vi "Migrate Measurements.vi"() -> ()   [LabVIEW 2021]
uses:
  _Measurement Plugin Converter/Migrator/Queue Driver/controls/Queue Operations.ctl
  _Measurement Plugin Converter/Migrator/Migration Logic/controls/Multiple Migration/Multiple Migration Data Holder.ctl
  <vilib>/Utility/sysdir.llb/System Directory Type.ctl
  <vilib>/Utility/miscctls.llb/LVRowAndColumnUnsignedTypeDef.ctl
  <vilib>/Utility/miscctls.llb/LVRowAndColumnTypeDef.ctl
  _Measurement Plugin Converter/Migrator/Migrator Reusables/controls/Dictionary States.ctl
  <vilib>/Utility/cursorutil.llb/Set Cursor (Icon Pict).vi
  _Measurement Plugin Converter/Migrator/Queue Driver/Queue Driver.lvlib
  _Measurement Plugin Converter/Migrator/Migration Logic/Migrator.lvlib
  _Measurement Plugin Converter/Migrator/Path Functions/Path Functions.lvlib
  _Measurement Plugin Converter/Migrator/Multiple Migrator/Multiple Migrator.lvlib
  _Measurement Plugin Converter/Migrator/Migrator Reusables/Migrator Reusables.lvlib
panel:
  out "error out":errorcluster
  in  "Tab Control":T1(tab)
  in  "Info":string
  in  "Select Measurement":path
  out "Warning":bool=TRUE caption="Warning:\nMeasurement should be an existing VI or folder path"
  in  "Populate measurements":bool
  in  "Select Project":path
  in  "Select all":bool
  in  "Back to Home":bool
  in  "List Plug-ins":bool
  in  "Select Measurements":string(tree)
  out "Selection warning":string="Atleast one measurement should be selected"
  out "Plug-in info":string="* Rename the Plug-in if required"
  out "Plug-in warning":string="Warning:\n1. Measurement plug-in name must be unique \n2. Plugin name cannot contain any of the following characters:\n         \\ / : * ? \" < > |"
  in  "Start Migration":bool
  in  "Back to Select":bool
  in  "List of Selected Measurements":i32(listbox)
  in  "Measurement Count":i32(slide)=6 caption="Migrating 1 of 1 measurement(s)" scale=0.0..100.0
  in  "Progress":i32(slide)=9 caption="Saving the project files..." scale=0.0..15.0
  in  "Review":bool
  in  "Migration Status":i32(listbox)
  in  "Back to Status":bool
  in  "Select Plug-in":string(combo) caption="Select Measurement plug-in to review"
  in  "Start Next":bool
  out "Launch Type Spec":string
  out "Launch Logic":string
  out "Launch UI":string
  # "* Project in which the measurement plug-in will be created"
  # "* Select a measurement vi or a folder containing measurements"
  # ".lvproj"
  # "Select the measurements to migrate"
  # "Review the Measurement:\n1. Review the Measurement UI. Click here to launch.\n2. Review the Measurement Logic VI. Click here to launch.\n3. Review the Type Specialization VI. Click here to launch."
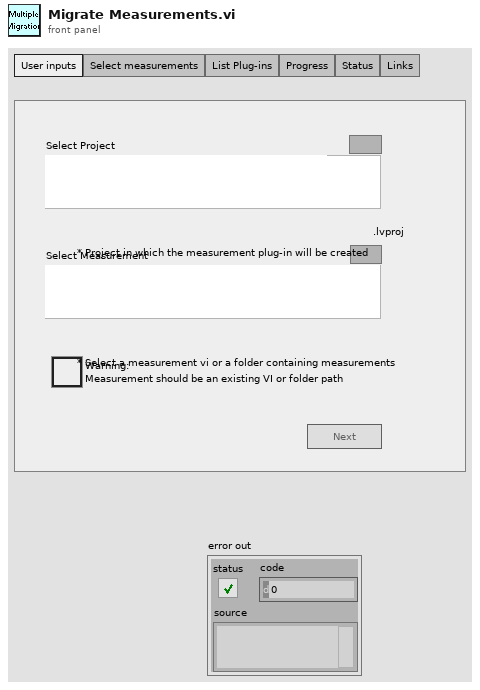
[diagram p1: front panel]
types:
  T1 = enum32{"User inputs", "Select measurements", "List Plug-ins", "Progress", "Status", "Links"}
  T2 = typedef "Queue Driver.lvlib/Queue Operations.ctl" = enum16{"Create Q", "Enqueue", "Enqueue N", "Dequeue", "Flush", "Release"}
  T3 = typedef "Migrator.lvlib/Multiple Migration Data Holder.ctl" = cluster{"Tree Reference":refnum<vi>, "LabVIEW Version":string, "Project path":path, "Create new project?":bool, "Measurement file/folder path":path, "Measurement folder selected?":bool, "Project warning":string, "Measurement warning":string, "Next clicked?":bool, "Measurement path changed?":bool, "Select all":bool, "Measurement folder Tags":string[], "Measurement file Tags":string[], "Selected cell Tag":string, "Measurement Plug-ins":string[][], "Measurement File Paths":path[], "Plugin Migration Value":i32, "Migration Count":i32, "Instrument containing subVIs":path[][], "Progress per measurement":i32, "Measurement Progress":i32, "Migration Status":string[][]}
  T4 = enum8{"Enabled", "Disabled", "Disabled and Grayed Out"}
  T5 = typedef "LVRowAndColumnUnsignedTypeDef.ctl" = cluster{"Row":u32, "Column":u32}
  T6 = typedef "LVRowAndColumnTypeDef.ctl" = cluster{"Row":i32, "Column":i32}
  T7 = typedef "Migrator Reusables.lvlib/Dictionary States.ctl" = enum16{"Set", "Get", "Delete", "Delete All"}
  T8 = typedef "System Directory Type.ctl" = i32
  T9 = typedef "LVPoint32TypeDef.ctl" = cluster{"Horizontal":i32, "Vertical":i32}
  T10 = typedef "Migrator.lvlib/Tree Items.ctl" = cluster{"Item name":string, "Indent":i32, "Tag":string}
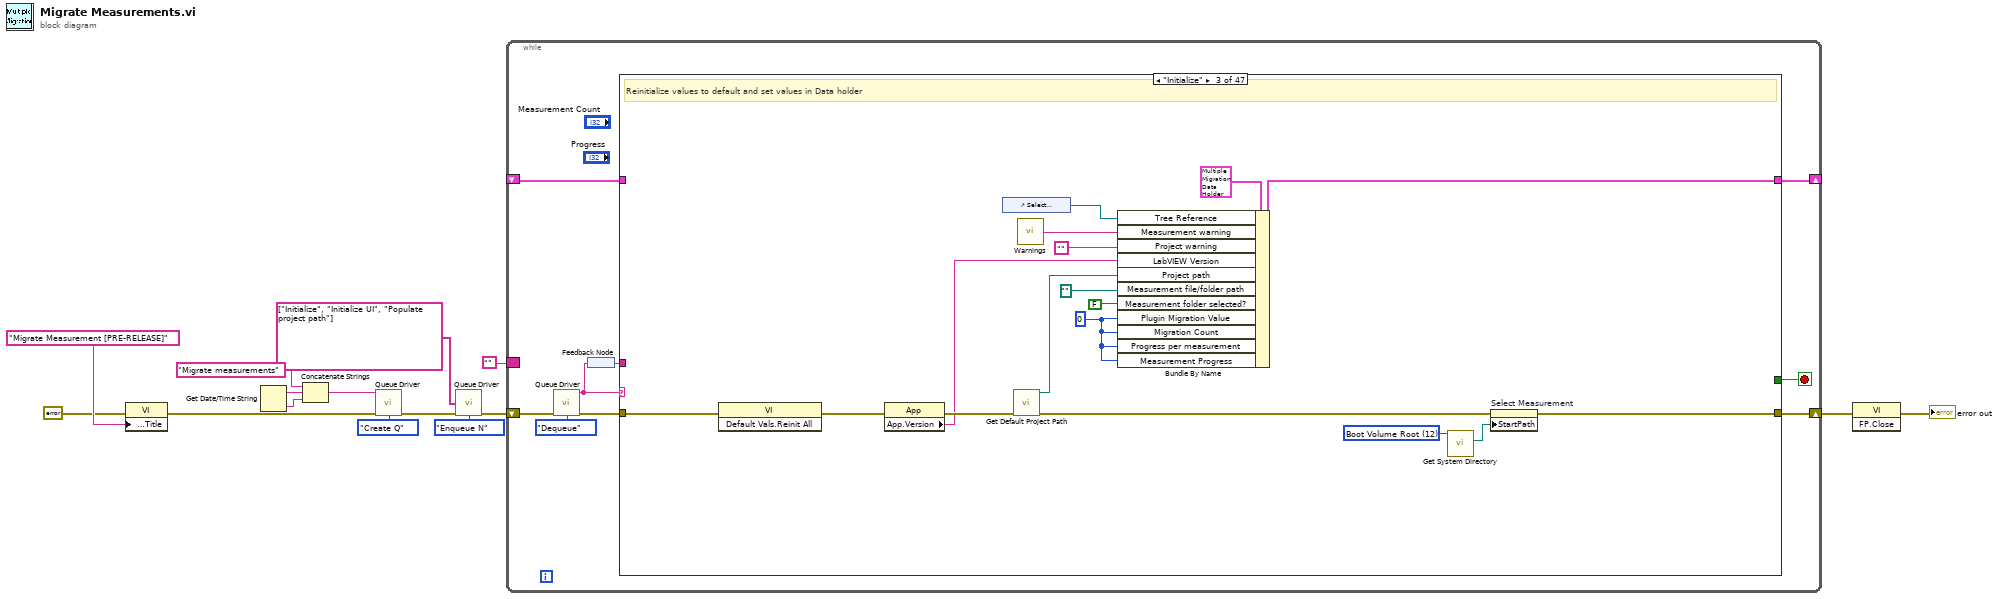
[diagram p0: block diagram]
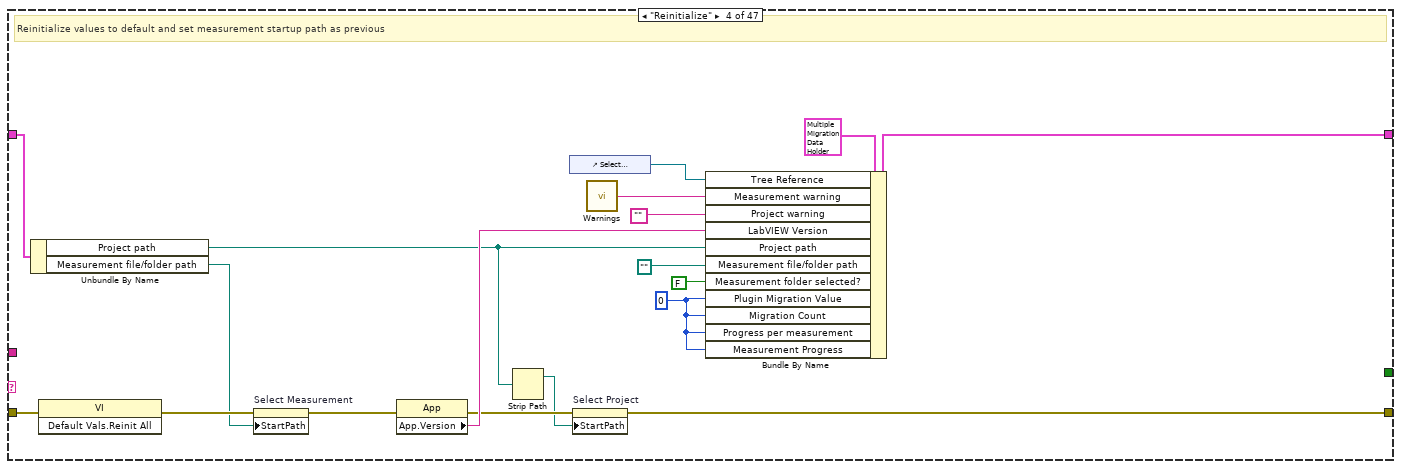
[diagram p4: hidden frame]
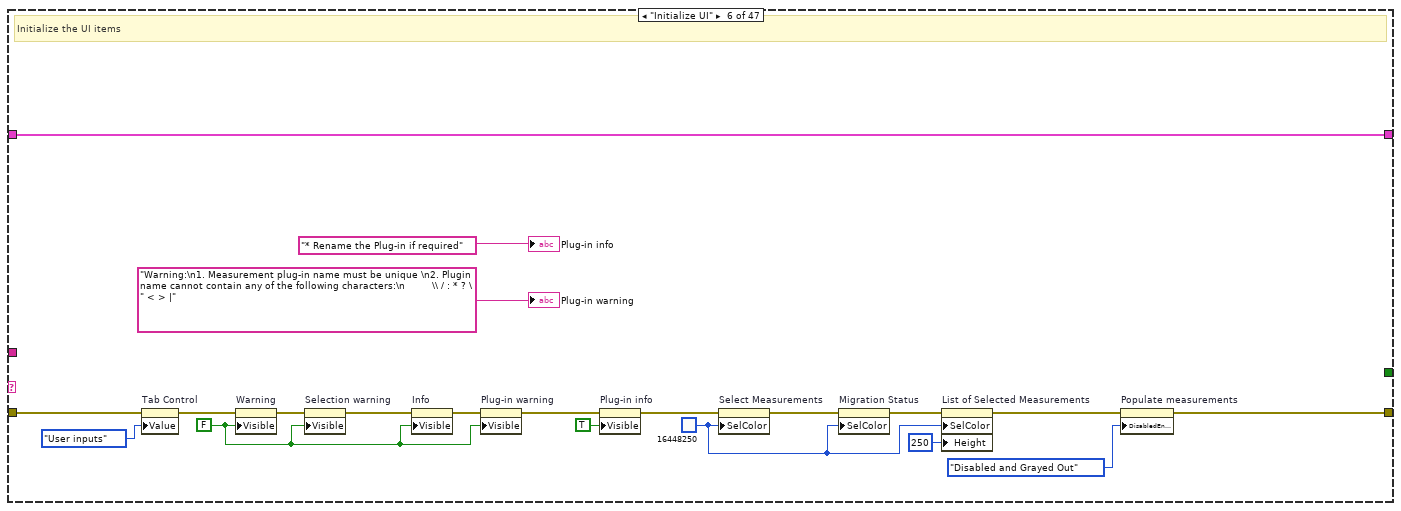
[diagram p6: hidden frame]
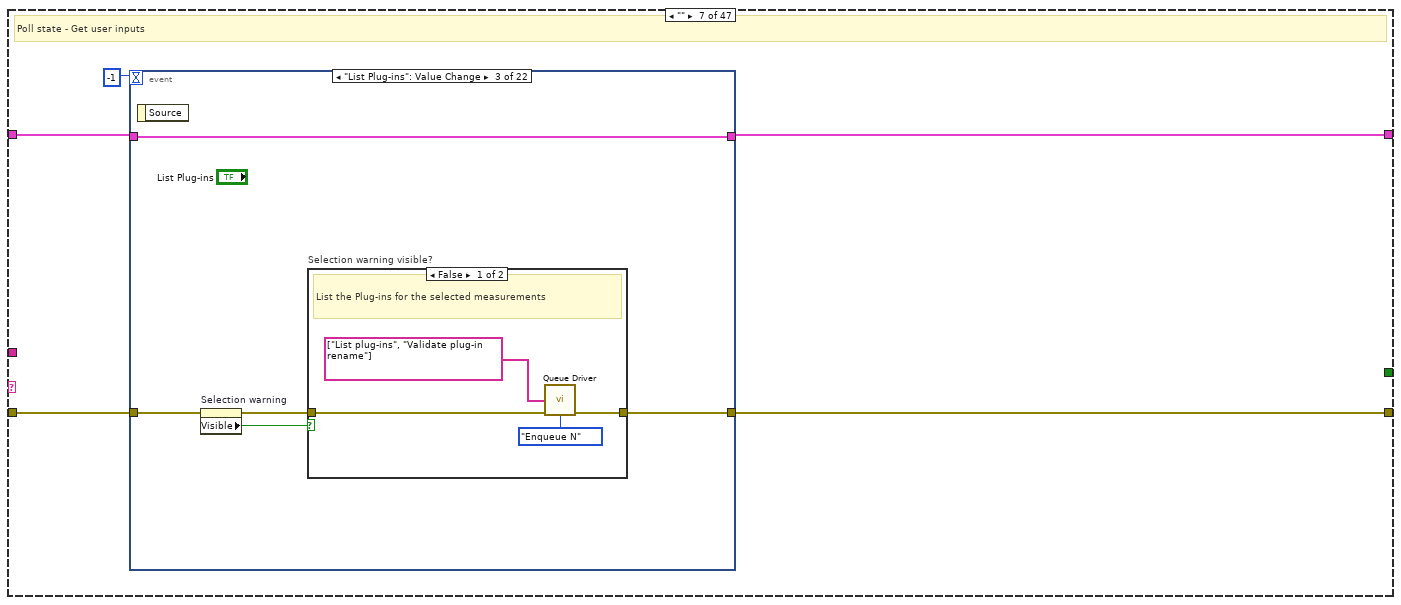
[diagram p7: hidden frame]
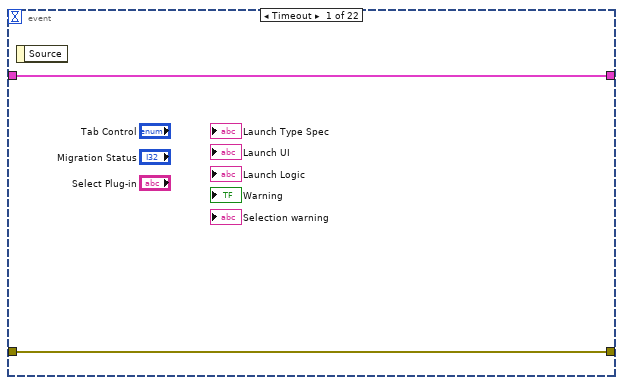
[diagram p8: hidden frame]
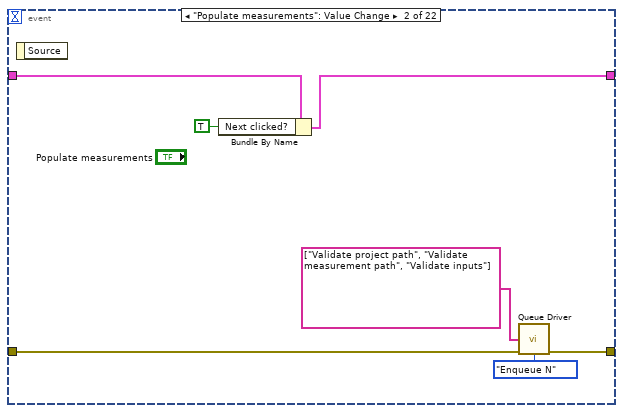
[diagram p9: hidden frame]
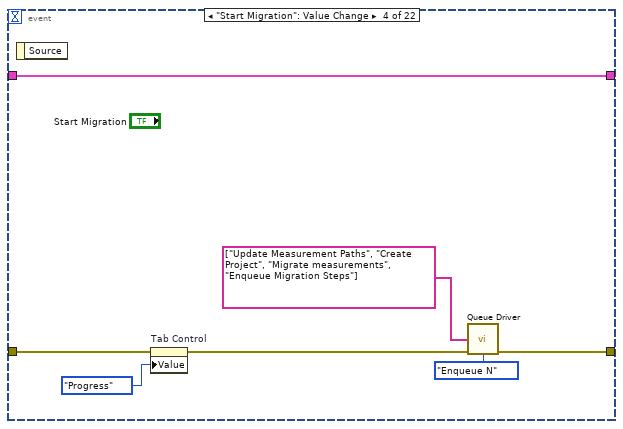
[diagram p11: hidden frame]
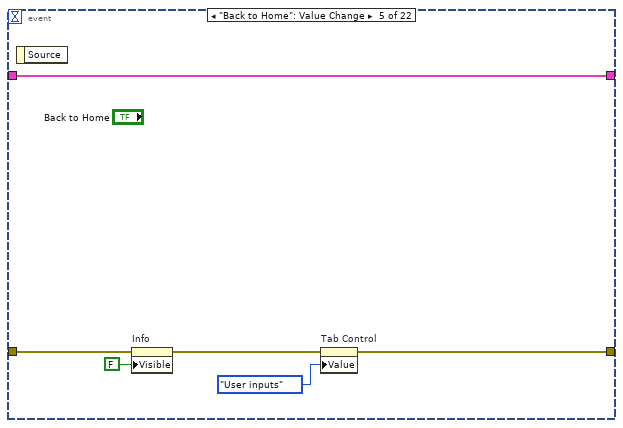
[diagram p12: hidden frame]
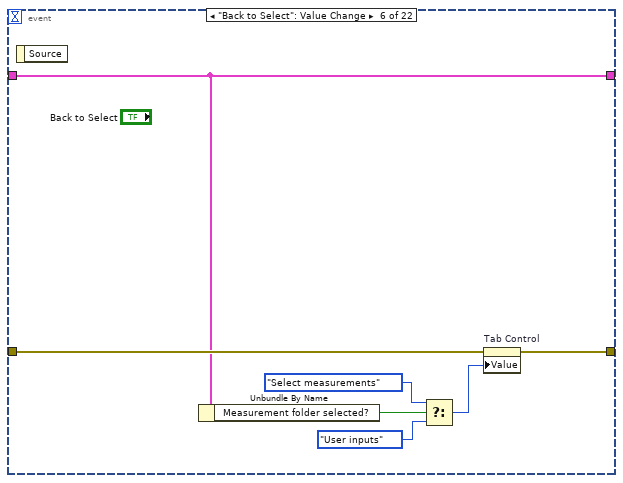
[diagram p13: hidden frame]
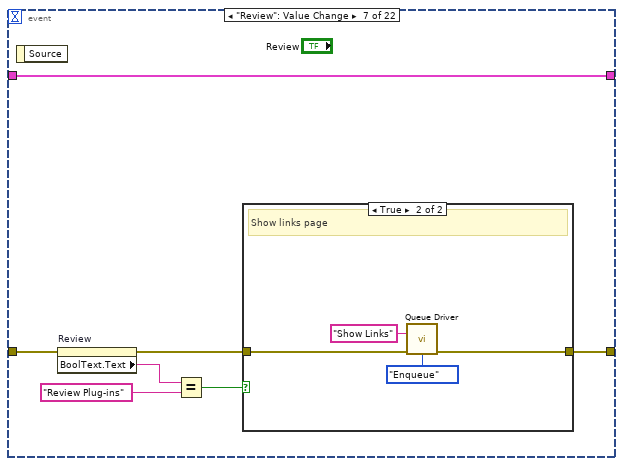
[diagram p14: hidden frame]
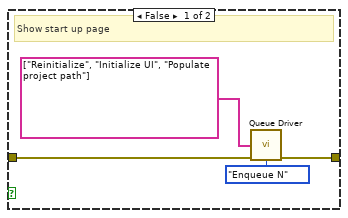
[diagram p15: hidden frame]
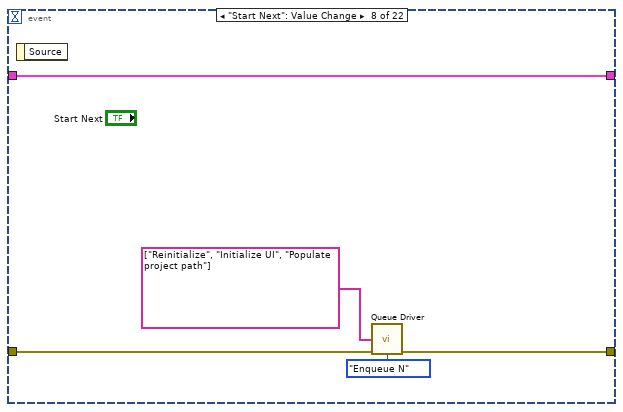
[diagram p16: hidden frame]
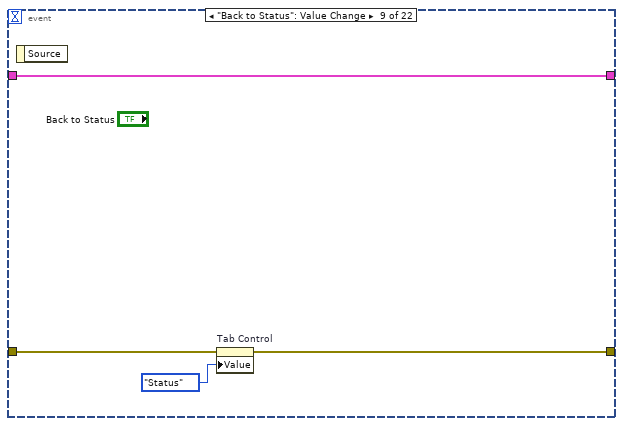
[diagram p17: hidden frame]
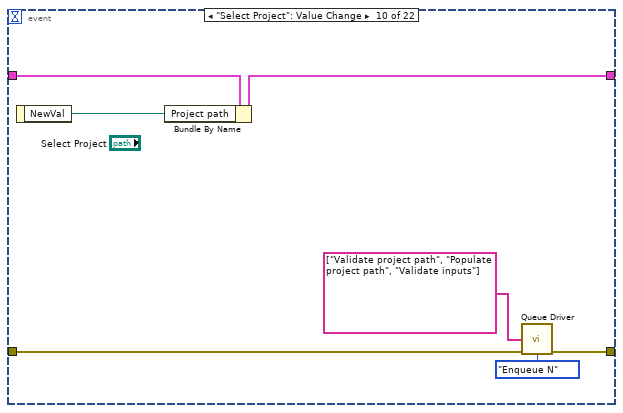
[diagram p18: hidden frame]
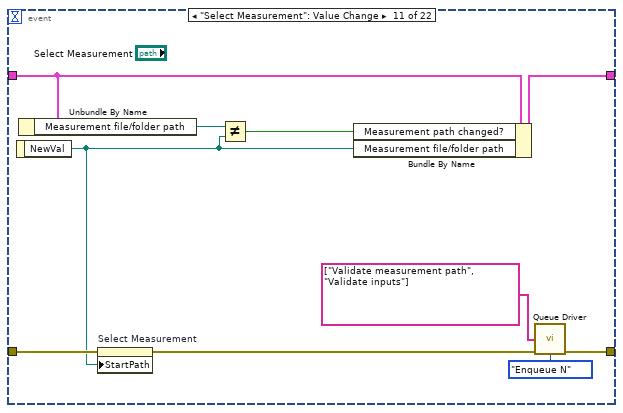
[diagram p19: hidden frame]
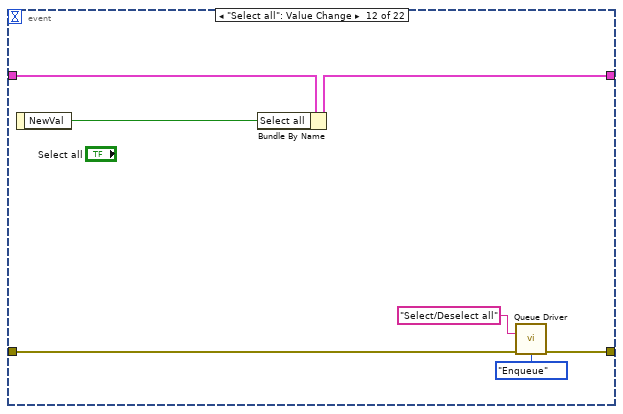
[diagram p20: hidden frame]
diagram:
  n1 = property class="VI"(error in=errorcluster {"status"=FALSE, "code"=0, "source"=""} ("error in (no error)"), "Front Panel.Title"="Migrate Measurement [PRE-RELEASE]" ("Front Panel Window:Title")) -> (error out=w1:errorcluster)  [unwired: 1 in, 1 out]
  n2 = Get Date/Time String() -> (date string=w12:string, time string=w11:string)  [unwired: 3 in]
  n3 = Concatenate Strings("Migrate measurements" ("string"), w12, w11) -> (w7:string)
  n4 = call "Queue Driver.vi"("Name"=w7, "error in (no error)"=w1, "Q Operations"=Queue_Operations."Create Q") -> ("error out"=w15:errorcluster)  [unwired: 11 in, 1 out]
  n5 = call "Queue Driver.vi"("States[]"=string[] ["Initialize", "Initialize UI", "Populate project path"], "error in (no error)"=w15, "Q Operations"=Queue_Operations."Enqueue N") -> ("error out"=w10:errorcluster)  [unwired: 11 in, 1 out]
  n6 = while {
    shift-right: [w23] -> w6
    shift-left: w10 -> [w24]
    shift-right: [w20] -> _
    shift-left: _ -> [w19]
    border: "" -> [_]
    stop <- w18 stop-if-true
    n7 = call "Queue Driver.vi"("error in (no error)"=w24, "Q Operations"=Queue_Operations."Dequeue") -> ("Dequeued State"=w17:string, "error out"=w22:errorcluster)  [unwired: 12 in]
    n8 = feedback #1() -> (w16:string)
    n9 = feedback-in #1(w17) -> ()
    n10 = case shown="\"Initialize\"" w17 {
      tunnel: w22 -> [w25 w28 w45 w63 w65 w85 w90 w262 w274 w285 w304 w328 w377 w394 w447 w472 w491 w548 w558 w564 w587 w597 w616 w633 w655 w662 w668 w674 w680 w686 w692 w698 w704 w710 w716 w722 w728 w734 w740 w762 w783 w795 w837 w846 w855 w876 w888]
      tunnel: [w25 w28 w34 w48 w65 w76 w89 w264 w274 w277 w303 w327 w377 w389 w435 w455 w478 w538 w558 w559 w584 w600 w615 w632 w654 w664 w670 w676 w682 w688 w694 w700 w706 w712 w718 w724 w730 w735 w744 w766 w783 w794 w834 w846 w852 w876 w878] -> w23
      tunnel: [w26 w27 w44 w62 w64 w81 w86 w263 w275 w280 w297 w315 w378 w395 w438 w470 w475 w543 w557 w579 w595 w609 w619 w652 w660 w666 w672 w678 w684 w690 w696 w702 w708 w714 w720 w726 w732 w738 w745 w767 w784 w799 w836 w847 w857 w877 w886] -> w20
      tunnel: w19 -> [w26 w27 _ w51 w64 w81 w87 w263 w275 w281 w299 w326 w378 w396 w439 w471 w476 w544 w557 w580 w595 w608 w619 w652 w660 w666 w672 w678 w684 w690 w696 w702 w708 w714 w720 w726 w732 w738 w746 w768 w784 w800 w836 w847 w857 w877 w886]
      tunnel: [_ _ _ _ _ _ _ _ _ _ _ _ _ _ _ _ _ _ _ _ _ _ _ _ _ _ _ _ _ _ _ _ _ _ _ _ _ _ _ _ _ _ _ _ _ _ TRUE] -> w18
      tunnel: w16 -> [_ _ _ _ _ _ _ _ _ _ _ _ _ _ _ _ _ _ _ _ _ _ _ _ _ _ _ _ _ _ _ _ _ _ _ _ _ _ _ _ _ _ _ _ w848 _ _]
      frame Default {
        # "Default case"
      }
      frame "/**********INITIALIZE**********/" {
      }
      frame "Initialize" {
        w29 = 0 ("Plugin Migration Value")
        w33 = T8 12 items=["User Home"=0, "User Desktop"=1, "User Documents"=2, "User Application Data"=3, "User Preferences"=4, "User Temporary"=5, "Public Documents"=6, "Public Application Data"=7, "Public Preferences"=8, "Public Cache"=13, "System Core Libraries"=9, "System Installed Libraries"=10, "Application Files"=11, "Boot Volume Root"=12] ("system directory type")
        # "Reinitialize values to default and set values in Data holder"
        n11 = invoke class="VI" method="Default Vals.Reinit All"(error in=w45) -> (error out=w42:errorcluster)  [unwired: 2 in, 2 out]
        n12 = property class="App"(error in=w42) -> (error out=w41:errorcluster, "App.Version"=w40:string)  [unwired: 1 in, 1 out]
        n13 = control-ref of="Select Measurements"() -> (w37:refnum<vi>)
        n14 = call "Get Default Project Path.vi"("error in"=w41) -> ("Project Path"=w43:path, "error out"=w35:errorcluster)  [unwired: 13 in]
        n15 = call "Warnings.vi"() -> ("Invalid measurement path"=w36:string)  [unwired: 8 in, 7 out]
        n16 = Bundle By Name(cluster=T3 {"Tree Reference"=refnum, "LabVIEW Version"="", "Project path"=path "", "Create new project?"=FALSE, "Measurement file/folder path"=path "", "Measurement folder selected?"=FALSE, "Project warning"="", "Measurement warning"="", "Next clicked?"=FALSE, "Measurement path changed?"=FALSE, "Select all"=FALSE, "Measurement folder Tags"=[], "Measurement file Tags"=[], "Selected cell Tag"="", "Measurement Plug-ins"=[], "Measurement File Paths"=[], "Plugin Migration Value"=0, "Migration Count"=0, "Instrument containing subVIs"=[], "Progress per measurement"=0, "Measurement Progress"=0, "Migration Status"=[]}, "Tree Reference"=w37, "Measurement warning"=w36, "Project warning"="", "LabVIEW Version"=w40, "Project path"=w43, "Measurement file/folder path"=path "", "Measurement folder selected?"=FALSE, "Plugin Migration Value"=w29, "Migration Count"=w29, "Progress per measurement"=w29, "Measurement Progress"=w29) -> (w44:T3)
        n17 = call <vilib>:"Get System Directory.vi"("system directory type"=w33) -> ("system directory"=w32:path)  [unwired: 10 in]
        n18 = property on="Select Measurement" class="Path"(error in=w35, "StartPath"=w32) -> (error out=w34:errorcluster)  [unwired: 1 in, 1 out]
      }
      frame "Reinitialize" {
        w54 = 0 ("Plugin Migration Value")
        # "Reinitialize values to default and set measurement startup path as previous"
        n19 = Unbundle By Name(w51) -> ("Project path"=w47:path, "Measurement file/folder path"=w50:path)
        n20 = invoke class="VI" method="Default Vals.Reinit All"(error in=w63) -> (error out=w53:errorcluster)  [unwired: 2 in, 2 out]
        n21 = property on="Select Measurement" class="Path"(error in=w53, "StartPath"=w50) -> (error out=w52:errorcluster)  [unwired: 1 in, 1 out]
        n22 = property class="App"(error in=w52) -> (error out=w49:errorcluster, "App.Version"=w61:string)  [unwired: 1 in, 1 out]
        n23 = Strip Path(path=w47) -> (stripped path=w46:path)  [unwired: 1 out]
        n24 = control-ref of="Select Measurements"() -> (w58:refnum<vi>)
        n25 = property on="Select Project" class="Path"(error in=w49, "StartPath"=w46) -> (error out=w48:errorcluster)  [unwired: 1 in, 1 out]
        n26 = call "Warnings.vi"() -> ("Invalid measurement path"=w57:string)  [unwired: 8 in, 7 out]
        n27 = Bundle By Name(cluster=T3 {"Tree Reference"=refnum, "LabVIEW Version"="", "Project path"=path "", "Create new project?"=FALSE, "Measurement file/folder path"=path "", "Measurement folder selected?"=FALSE, "Project warning"="", "Measurement warning"="", "Next clicked?"=FALSE, "Measurement path changed?"=FALSE, "Select all"=FALSE, "Measurement folder Tags"=[], "Measurement file Tags"=[], "Selected cell Tag"="", "Measurement Plug-ins"=[], "Measurement File Paths"=[], "Plugin Migration Value"=0, "Migration Count"=0, "Instrument containing subVIs"=[], "Progress per measurement"=0, "Measurement Progress"=0, "Migration Status"=[]}, "Tree Reference"=w58, "Measurement warning"=w57, "Project warning"="", "LabVIEW Version"=w61, "Project path"=w47, "Measurement file/folder path"=path "", "Measurement folder selected?"=FALSE, "Plugin Migration Value"=w54, "Migration Count"=w54, "Progress per measurement"=w54, "Measurement Progress"=w54) -> (w62:T3)
      }
      frame "/**********FP RELATED**********/" {
      }
      frame "Initialize UI" {
        w70 = FALSE ("Visible")
        w78 = u32 16448250 ("Selection Color")
        # "Initialize the UI items"
        n28 = property on="Tab Control" class="TabCtl (strict)"(error in=w85, "Value"=T1."User inputs" ("Tab Control")) -> (error out=w80:errorcluster)  [unwired: 1 in, 1 out]
        n29 = property on="Warning" class="Bool"(error in=w80, "Visible"=w70) -> (error out=w79:errorcluster)  [unwired: 1 in, 1 out]
        n30 = property on="Selection warning" class="Str"(error in=w79, "Visible"=w70) -> (error out=w74:errorcluster)  [unwired: 1 in, 1 out]
        n31 = property on="Info" class="Str"(error in=w74, "Visible"=w70) -> (error out=w73:errorcluster)  [unwired: 1 in, 1 out]
        n32 = property on="Plug-in warning" class="Str"(error in=w73, "Visible"=w70) -> (error out=w69:errorcluster)  [unwired: 1 in, 1 out]
        n33 = property on="Plug-in info" class="Str"(error in=w69, "Visible"=TRUE) -> (error out=w68:errorcluster)  [unwired: 1 in, 1 out]
        n34 = property on="Select Measurements" class="Tree (strict)"(error in=w68, "SelColor"=w78) -> (error out=w83:errorcluster)  [unwired: 1 in, 1 out]
        n35 = property on="Migration Status" class="MCListbox (strict)"(error in=w83, "SelColor"=w78) -> (error out=w82:errorcluster)  [unwired: 1 in, 1 out]
        n36 = property on="List of Selected Measurements" class="MCListbox (strict)"(error in=w82, "SelColor"=w78, "Height"=u32 250 ("Size:Height")) -> (error out=w77:errorcluster)  [unwired: 1 in, 1 out]
        n37 = property on="Populate measurements" class="Bool"(error in=w77, "DisabledEnum"=T4."Disabled and Grayed Out" ("Disabled")) -> (error out=w76:errorcluster)  [unwired: 1 in, 1 out]
        "Plug-in warning" <- "Warning:\n1. Measurement plug-in name must be unique \n2. Plugin name cannot contain any of the following characters:\n         \\ / : * ? \" < > |" ("f")
        "Plug-in info" <- "* Rename the Plug-in if required" ("Plug-in warning")
      }
      frame "" {
        # "Poll state - Get user inputs"
        n38 = event shown="[2] \"List Plug-ins\": Value Change" {
          selector: _ -> [_ _ _ _ _ _ _ _ _ _ _ _ _ _ _ _ _ _ _ _ _ _]
          dyn-events: _ -> [_ _ _ _ _ _ _ _ _ _ _ _ _ _ _ _ _ _ _ _ _ _]
          timeout: -1 -> [_ _ _ _ _ _ _ _ _ _ _ _ _ _ _ _ _ _ _ _ _ _]
          tunnel: w90 -> [w92 w99 w102 w116 w119 w129 w133 w146 w153 w160 w166 w174 w185 w194 w202 w209 w212 w216 w222 w232 w244 w256]
          tunnel: [w92 w98 w103 w112 w122 w128 w135 w147 w152 w159 w169 w173 w180 w193 w200 w210 w213 w217 w224 w235 w246 w255] -> w89
          tunnel: w87 -> [w91 w95 w104 w113 w120 w127 w136 w149 w150 w157 w164 w177 w184 w195 w203 w211 w215 w219 w225 w236 w247 w257]
          tunnel: [w91 w94 w104 w113 w120 w127 w136 w149 w150 w156 w170 w176 w183 w195 w203 w211 w215 w219 w225 w236 w247 w257] -> w86
          event Timeout {
            # "Timeout"
            n39 = event-data() -> ()  [unwired: 1 in, 1 out]
          }
          event "Populate measurements": Value Change {
            n40 = event-data() -> ()  [unwired: 1 in, 1 out]
            n41 = Bundle By Name(cluster=w95, "Next clicked?"=TRUE) -> (w94:T3)
            n42 = call "Queue Driver.vi"("States[]"=string[] ["Validate project path", "Validate measurement path", "Validate inputs"], "error in (no error)"=w99, "Q Operations"=Queue_Operations."Enqueue N") -> ("error out"=w98:errorcluster)  [unwired: 11 in, 1 out]
          }
          event "List Plug-ins": Value Change {
            n43 = event-data() -> ()  [unwired: 1 in, 1 out]
            n44 = property on="Selection warning" class="Str"(error in=w102) -> (error out=w101:errorcluster, "Visible"=w100:bool)  [unwired: 1 in, 1 out]
            n45 = case "Selection warning visible?" shown="False" w100 {
              tunnel: w101 -> [w108 w109]
              tunnel: [w107 w109] -> w103
              frame False {
                # "List the Plug-ins for the selected measurements"
                n46 = call "Queue Driver.vi"("States[]"=string[] ["List plug-ins", "Validate plug-in rename"], "error in (no error)"=w108, "Q Operations"=Queue_Operations."Enqueue N") -> ("error out"=w107:errorcluster)  [unwired: 11 in, 1 out]
              }
              frame True {
                # "Pass"
              }
            }
          }
          event "Start Migration": Value Change {
            n47 = event-data() -> ()  [unwired: 1 in, 1 out]
            n48 = property on="Tab Control" class="TabCtl (strict)"(error in=w116, "Value"=T1."Progress" ("Tab Control")) -> (error out=w115:errorcluster)  [unwired: 1 in, 1 out]
            n49 = call "Queue Driver.vi"("States[]"=string[] ["Update Measurement Paths", "Create Project", "Migrate measurements", "Enqueue Migration Steps"], "error in (no error)"=w115, "Q Operations"=Queue_Operations."Enqueue N") -> ("error out"=w112:errorcluster)  [unwired: 11 in, 1 out]
          }
          event "Back to Home": Value Change {
            n50 = event-data() -> ()  [unwired: 1 in, 1 out]
            n51 = property on="Info" class="Str"(error in=w119, "Visible"=FALSE) -> (error out=w118:errorcluster)  [unwired: 1 in, 1 out]
            n52 = property on="Tab Control" class="TabCtl (strict)"(error in=w118, "Value"=T1."User inputs" ("Tab Control")) -> (error out=w122:errorcluster)  [unwired: 1 in, 1 out]
          }
          event "Back to Select": Value Change {
            n53 = event-data() -> ()  [unwired: 1 in, 1 out]
            n54 = Unbundle By Name(w127) -> ("Measurement folder selected?"=w126:bool)
            n55 = Select(t=T1."Select measurements" ("Tab Control"), s=w126, f=T1."User inputs" ("Tab Control")) -> (s? t:f=w123:T1)
            n56 = property on="Tab Control" class="TabCtl (strict)"(error in=w129, "Value"=w123) -> (error out=w128:errorcluster)  [unwired: 1 in, 1 out]
          }
          event "Review": Value Change {
            n57 = event-data() -> ()  [unwired: 1 in, 1 out]
            n58 = property on="Review" class="Bool"(error in=w133) -> (error out=w134:errorcluster, "BoolText.Text"=w132:string)  [unwired: 1 in, 1 out]
            n59 = Equal?(x=w132, y="Review Plug-ins") -> (x = y?=w130:bool)
            n60 = case shown="True" w130 {
              tunnel: [w138 w144] -> w135
              tunnel: w134 -> [w137 w141]
              frame False {
                # "Show start up page"
                n61 = call "Queue Driver.vi"("States[]"=string[] ["Reinitialize", "Initialize UI", "Populate project path"], "error in (no error)"=w137, "Q Operations"=Queue_Operations."Enqueue N") -> ("error out"=w138:errorcluster)  [unwired: 11 in, 1 out]
              }
              frame True {
                # "Show links page"
                n62 = call "Queue Driver.vi"("State"="Show Links", "error in (no error)"=w141, "Q Operations"=Queue_Operations."Enqueue") -> ("error out"=w144:errorcluster)  [unwired: 11 in, 1 out]
              }
            }
          }
          event "Start Next": Value Change {
            n63 = event-data() -> ()  [unwired: 1 in, 1 out]
            n64 = call "Queue Driver.vi"("States[]"=string[] ["Reinitialize", "Initialize UI", "Populate project path"], "error in (no error)"=w146, "Q Operations"=Queue_Operations."Enqueue N") -> ("error out"=w147:errorcluster)  [unwired: 11 in, 1 out]
          }
          event "Back to Status": Value Change {
            n65 = event-data() -> ()  [unwired: 1 in, 1 out]
            n66 = property on="Tab Control" class="TabCtl (strict)"(error in=w153, "Value"=T1."Status" ("Tab Control")) -> (error out=w152:errorcluster)  [unwired: 1 in, 1 out]
          }
          event "Select Project": Value Change {
            n67 = event-data() -> ("NewVal"=w155:path)  [unwired: 1 in]
            n68 = Bundle By Name(cluster=w157, "Project path"=w155) -> (w156:T3)
            n69 = call "Queue Driver.vi"("States[]"=string[] ["Validate project path", "Populate project path", "Validate inputs"], "error in (no error)"=w160, "Q Operations"=Queue_Operations."Enqueue N") -> ("error out"=w159:errorcluster)  [unwired: 11 in, 1 out]
          }
          event "Select Measurement": Value Change {
            n70 = event-data() -> ("NewVal"=w161:path)  [unwired: 1 in]
            n71 = Unbundle By Name(w164) -> ("Measurement file/folder path"=w162:path)
            n72 = property on="Select Measurement" class="Path"(error in=w166, "StartPath"=w161) -> (error out=w165:errorcluster)  [unwired: 1 in, 1 out]
            n73 = Not Equal?(x=w162, y=w161) -> (x != y?=w163:bool)
            n74 = Bundle By Name(cluster=w164, "Measurement path changed?"=w163, "Measurement file/folder path"=w161) -> (w170:T3)
            n75 = call "Queue Driver.vi"("States[]"=string[] ["Validate measurement path", "Validate inputs"], "error in (no error)"=w165, "Q Operations"=Queue_Operations."Enqueue N") -> ("error out"=w169:errorcluster)  [unwired: 11 in, 1 out]
          }
          event "Select all": Value Change {
            n76 = event-data() -> ("NewVal"=w175:bool)  [unwired: 1 in]
            n77 = Bundle By Name(cluster=w177, "Select all"=w175) -> (w176:T3)
            n78 = call "Queue Driver.vi"("State"="Select/Deselect all", "error in (no error)"=w174, "Q Operations"=Queue_Operations."Enqueue") -> ("error out"=w173:errorcluster)  [unwired: 11 in, 1 out]
          }
          event "Select Measurements": Mouse Down {
            n79 = event-data() -> ("Coords"=w178:T9)  [unwired: 1 in]
            n80 = invoke on="Select Measurements" class="Tree (strict)" method="Point To Row Column"(error in=w185, "Point"=w178) -> (error out=w181:errorcluster, "Tag"=w182:string, "InGlyph"=w179:bool)  [unwired: 6 in, 5 out]
            n81 = case "In Symbol?" shown="True" w179 {
              tunnel: w181 -> [w186 w190]
              tunnel: [w186 w189] -> w180
              frame False {
                # "Pass"
              }
              frame True {
                # "Update the selection of measurements"
                n82 = call "Queue Driver.vi"("State"="Measurement selection" ("State 2"), "error in (no error)"=w190, "Q Operations"=Queue_Operations."Enqueue") -> ("error out"=w189:errorcluster)  [unwired: 11 in, 1 out]
              }
            }
            n83 = Bundle By Name(cluster=w184, "Selected cell Tag"=w182) -> (w183:T3)
          }
          event "List of Selected Measurements": Edit Cell {
            n84 = event-data() -> ()  [unwired: 1 in, 1 out]
            n85 = call "Queue Driver.vi"("State"="Validate plug-in rename", "error in (no error)"=w194, "Q Operations"=Queue_Operations."Enqueue") -> ("error out"=w193:errorcluster)  [unwired: 11 in, 1 out]
          }
          event "List of Selected Measurements": Mouse Down {
            n86 = event-data() -> ("Coords"=w199:T9)  [unwired: 1 in, 7 out]
            n87 = invoke on="List of Selected Measurements" class="MCListbox (strict)" method="Point To Row Column"(error in=w202, "Point"=w199) -> (error out=w201:errorcluster, "CellPosition"=w196:T6)  [unwired: 5 in, 5 out]
            n88 = Unbundle By Name(w196) -> ("Column"=w198:i32)
            n89 = Not Equal To 0?(x=w198) -> (x != 0?=w197:bool)
            n90 = case shown="False" w197 {
              tunnel: w201 -> [w204 w207]
              tunnel: [w204 w206] -> w200
              tunnel: w196 -> [_ w205]
              frame False {
              }
              frame True {
                n91 = property on="List of Selected Measurements" class="MCListbox (strict)"(error in=w207, "EditPos"=w205) -> (error out=w206:errorcluster)  [unwired: 1 in, 1 out]
              }
            }
          }
          event "Select Plug-in": Value Change {
            n92 = event-data() -> ("NewVal"=w208:string)  [unwired: 1 in]
            n93 = call "Set Measurement Name.vi"("Name"=w208, "error in (no error)"=w209) -> ("error out"=w210:errorcluster)  [unwired: 13 in]
          }
          event "Launch UI", "Launch Logic", "Launch Type Spec": Mouse Enter {
            n94 = event-data() -> ()  [unwired: 1 in, 1 out]
            n95 = call-poly <vilib>:"Set Cursor.vi"("error in (no error)"=w212, "icon"=u16 6) -> ("error out"=w213:errorcluster)  [unwired: 8 in, 1 out]
          }
          event "Launch UI", "Launch Logic", "Launch Type Spec": Mouse Leave {
            n96 = event-data() -> ()  [unwired: 1 in, 1 out]
            n97 = call-poly <vilib>:"Set Cursor.vi"("error in (no error)"=w216, "icon"=u16 0) -> ("error out"=w217:errorcluster)  [unwired: 8 in, 1 out]
          }
          event "Launch UI": Mouse Down {
            n98 = event-data() -> ()  [unwired: 1 in, 1 out]
            n99 = property on="Select Plug-in" class="CmbBox"(error in=w222) -> (error out=w223:errorcluster, "Value"=w221:string)  [unwired: 1 in, 1 out]
            n100 = Empty String/Path?(string/path=w221) -> (empty?=w220:bool)
            n101 = case shown="False" w220 {
              tunnel: [w228 w230] -> w224
              tunnel: w223 -> [w226 w230]
              frame False {
                n102 = call "Measurement Plugin Path.vi"("error in (no error)"=w226) -> ("Measurement UI"=w227:path, "error out"=w229:errorcluster)  [unwired: 2 in, 11 out]
                n103 = call "Open VI.vi"("Logic VI Path"=w227, "error in (no error)"=w229) -> ("error out"=w228:errorcluster)  [unwired: 13 in]
              }
              frame True {
              }
            }
          }
          event "Launch Logic": Mouse Down {
            n104 = event-data() -> ()  [unwired: 1 in, 1 out]
            n105 = property on="Select Plug-in" class="CmbBox"(error in=w232) -> (error out=w233:errorcluster, "Value"=w234:string)  [unwired: 1 in, 1 out]
            n106 = Empty String/Path?(string/path=w234) -> (empty?=w231:bool)
            n107 = case shown="False" w231 {
              tunnel: [w239 w241] -> w235
              tunnel: w233 -> [w238 w241]
              frame False {
                n108 = call "Measurement Plugin Path.vi"("error in (no error)"=w238) -> ("Logic VI Path"=w237:path, "error out"=w240:errorcluster)  [unwired: 2 in, 11 out]
                n109 = call "Open VI.vi"("Logic VI Path"=w237, "error in (no error)"=w240) -> ("error out"=w239:errorcluster)  [unwired: 13 in]
              }
              frame True {
              }
            }
          }
          event "Launch Type Spec": Mouse Down {
            n110 = event-data() -> ()  [unwired: 1 in, 1 out]
            n111 = property on="Select Plug-in" class="CmbBox"(error in=w244) -> (error out=w243:errorcluster, "Value"=w245:string)  [unwired: 1 in, 1 out]
            n112 = Empty String/Path?(string/path=w245) -> (empty?=w242:bool)
            n113 = case shown="False" w242 {
              tunnel: [w250 w252] -> w246
              tunnel: w243 -> [w249 w252]
              frame False {
                n114 = call "Measurement Plugin Path.vi"("error in (no error)"=w249) -> ("Type Specialization"=w248:path, "error out"=w251:errorcluster)  [unwired: 2 in, 11 out]
                n115 = call "Open VI.vi"("Logic VI Path"=w248, "error in (no error)"=w251) -> ("error out"=w250:errorcluster)  [unwired: 13 in]
              }
              frame True {
              }
            }
          }
          event Panel Close? {
            n116 = event-data() -> ()  [unwired: 1 in, 1 out]
            n117 = call "Queue Driver.vi"("State"="Exit", "error in (no error)"=w256, "Q Operations"=Queue_Operations."Enqueue") -> ("error out"=w255:errorcluster)  [unwired: 11 in, 1 out]
            n118 = event-data("Discard?"=TRUE) -> ()  [unwired: 1 in, 1 out]
          }
        }
      }
      frame "Populate project path" {
        # "Populate the validated project path in the control"
        n119 = Unbundle By Name(w263) -> ("Project warning"=w260:string, "Project path"=w261:path)
        n120 = Empty String/Path?(string/path=w260) -> (empty?=w259:bool)
        n121 = case "Valid project?" shown="True" w259 {
          tunnel: [w265 w273] -> w264
          tunnel: w262 -> [w265 w272]
          tunnel: w261 -> [_ w267]
          frame False {
            # "Pass"
          }
          frame True {
            # "Populate the path in the control"
            n122 = call <vilib>:"Get File Extension.vi"("error in (no error)"=w272, "file"=w267) -> ("error out"=w271:errorcluster, "filename without extension"=w270:string)  [unwired: 5 in, 3 out]
            n123 = Concatenate Strings("..\\" ("string"), w270) -> (w268:string)
            n124 = Build Path(base path=w267, name or relative path=w268) -> (appended path=w266:path)
            n125 = property on="Select Project" class="Path"(error in=w271, "Value"=w266) -> (error out=w273:errorcluster)  [unwired: 1 in, 1 out]
          }
        }
      }
      frame "/**********INPUT VALIDATION**********/" {
      }
      frame "Validate project path" {
        # "Validate the project path and set warning if required"
        n126 = Unbundle By Name(w281) -> ("Project path"=w282:path, "LabVIEW Version"=w283:string)
        n127 = call <vilib>:"Is Path and Not Empty.vi"("path"=w282) -> ("Is Path and Not Empty?"=w284:bool)  [unwired: 4 in]
        n128 = case "Is Path and not empty?" shown="True" w284 {
          tunnel: w285 -> [w288 w295]
          tunnel: [w288 w294] -> w277
          tunnel: [w286 w293] -> w276
          tunnel: w283 -> [_ w292]
          tunnel: w282 -> [w287 w291]
          tunnel: [_ w290] -> w279
          tunnel: [w287 w289] -> w278
          frame False {
            # "Set warning"
            n129 = call "Warnings.vi"() -> ("Invalid project path"=w286:string)  [unwired: 8 in, 7 out]
          }
          frame True {
            # "Validate the path"
            n130 = call "Validate Project Path.vi"("Project path in"=w291, "LabVIEW Version"=w292, "error in (no error)"=w295) -> ("Validated project path"=w289:path, "New project?"=w290:bool, "Warning"=w293:string, "error out"=w294:errorcluster)  [unwired: 9 in]
          }
        }
        n131 = Bundle By Name(cluster=w281, "Project path"=w278, "Create new project?"=w279, "Project warning"=w276) -> (w280:T3)
      }
      frame "Validate measurement path" {
        # "Validate the measurement path and set warning if required"
        n132 = Unbundle By Name(w299) -> ("Measurement file/folder path"=w301:path, "LabVIEW Version"=w302:string)
        n133 = call <vilib>:"Is Path and Not Empty.vi"("path"=w301) -> ("Is Path and Not Empty?"=w300:bool)  [unwired: 4 in]
        n134 = case "Is Path and not empty?" shown="True" w300 {
          tunnel: w304 -> [w306 w312]
          tunnel: w301 -> [_ w311]
          tunnel: w302 -> [_ w310]
          tunnel: [w306 w309] -> w303
          tunnel: [w305 w308] -> w296
          tunnel: [_ w307] -> w298
          frame False {
            # "Set warning"
            n135 = call "Warnings.vi"() -> ("Invalid measurement path"=w305:string)  [unwired: 8 in, 7 out]
          }
          frame True {
            # "Validate the path"
            n136 = call "Validate Measurement Path.vi"("Measurement path"=w311, "LabVIEW version"=w310, "error in (no error)"=w312) -> ("Folder?"=w307:bool, "Warning"=w308:string, "error out"=w309:errorcluster)  [unwired: 10 in]
          }
        }
        n137 = Bundle By Name(cluster=w299, "Measurement folder selected?"=w298, "Measurement warning"=w296) -> (w297:T3)
      }
      frame "Validate inputs" {
        # "Validate the project path and measurement path inputs"
        n138 = Unbundle By Name(w326) -> ("Project warning"=w320:string, "Measurement warning"=w325:string, "Next clicked?"=w321:bool, "Project warning"=w319:string, "Measurement warning"=w318:string, "Measurement folder selected?"=w317:bool, "Measurement path changed?"=w316:bool)
        n139 = Empty String/Path?(string/path=w325) -> (empty?=w324:bool)
        n140 = Empty String/Path?(string/path=w320) -> (empty?=w323:bool)
        n141 = And(x=w323, y=w324) -> (x .and. y?=w322:bool)
        n142 = case "Valid inputs?" shown="True" w322 {
          tunnel: w328 -> [w342 w352]
          tunnel: [w337 w348] -> w327
          tunnel: w321 -> [_ w346]
          tunnel: w319 -> [w330 _]
          tunnel: w318 -> [w333 _]
          tunnel: w317 -> [_ w345]
          tunnel: w316 -> [w329 w344]
          tunnel: [w329 w343] -> w313
          frame False {
            # "Set the appropriate warning"
            n143 = call "Edit Warning.vi"("Warning in"=w330) -> ("Warning out"=w332:string)  [unwired: 6 in]
            n144 = call "Edit Warning.vi"("Warning in"=w333) -> ("Warning out"=w331:string)  [unwired: 6 in]
            n145 = Concatenate Strings("Warning:" ("string"), "\n", w332, w331) -> (w335:string)
            n146 = call "Get Warning Position.vi"("Warning"=w335) -> ("Warning position"=w334:i32)  [unwired: 6 in]
            n147 = property on="Warning" class="Bool"(error in=w342, "Visible"=TRUE, "Caption.Text"=w335, "Caption.Top"=w334) -> (error out=w338:errorcluster)  [unwired: 1 in, 1 out]
            n148 = property on="Populate measurements" class="Bool"(error in=w338, "DisabledEnum"=T4."Disabled and Grayed Out" ("Disabled")) -> (error out=w337:errorcluster)  [unwired: 1 in, 1 out]
          }
          frame True {
            # "Check if next is clicked and make the warning invisible"
            n149 = case "Next clicked?" shown="True" w346 {
              tunnel: w352 -> [w354 w359]
              tunnel: [w354 w358] -> w351
              tunnel: w345 -> [_ w357]
              tunnel: w344 -> [w353 w356]
              tunnel: [w353 FALSE] -> w343
              frame False {
                # "Pass"
              }
              frame True {
                # "Populate measurements if folder is selected and List the plug-ins if not"
                n150 = case "Measurement path changed?" shown="True" w356 {
                  tunnel: w359 -> [w365 w368]
                  tunnel: [w364 w367] -> w358
                  tunnel: w357 -> [w360 w366]
                  frame False {
                    # "Measurement folder?"
                    n151 = Select(t=T1."Select measurements" ("Tab Control"), s=w360, f=T1."List Plug-ins" ("Tab Control")) -> (s? t:f=w361:T1)
                    n152 = property on="Tab Control" class="TabCtl (strict)"(error in=w365, "Value"=w361) -> (error out=w364:errorcluster)  [unwired: 1 in, 1 out]
                  }
                  frame True {
                    n153 = case "Measurement folder?" shown="True" w366 {
                      tunnel: w368 -> [w372 w376]
                      tunnel: [w371 w375] -> w367
                      frame True {
                        n154 = call "Queue Driver.vi"("State"="Populate measurements" ("State 2"), "error in (no error)"=w372, "Q Operations"=Queue_Operations."Enqueue") -> ("error out"=w371:errorcluster)  [unwired: 11 in, 1 out]
                      }
                      frame False {
                        n155 = call "Queue Driver.vi"("States[]"=string[] ["List plug-ins", "Validate plug-in rename"], "error in (no error)"=w376, "Q Operations"=Queue_Operations."Enqueue N") -> ("error out"=w375:errorcluster)  [unwired: 11 in, 1 out]
                      }
                    }
                  }
                }
              }
            }
            n156 = property on="Warning" class="Bool"(error in=w351, "Visible"=FALSE) -> (error out=w349:errorcluster)  [unwired: 1 in, 1 out]
            n157 = property on="Populate measurements" class="Bool"(error in=w349, "DisabledEnum"=T4."Enabled" ("Disabled")) -> (error out=w348:errorcluster)  [unwired: 1 in, 1 out]
          }
        }
        n158 = Bundle By Name(cluster=w326, "Next clicked?"=FALSE, "Measurement path changed?"=w313) -> (w315:T3)
      }
      frame "/**********FUNCTIONALITY**********/" {
      }
      frame "Populate measurements" {
        w383 = TRUE ("Visible")
        # "Populate the measurements in the Tree and set icon to the items"
        n159 = Unbundle By Name(w396) -> ("Tree Reference"=w390:refnum<vi>, "Measurement file/folder path"=w399:path, "LabVIEW Version"=w397:string)
        n160 = call "Set Cursor Icon.vi"("Cursor icon"=u16 2, "error in (no error)"=w394) -> ("error out"=w393:errorcluster)  [unwired: 13 in]
        n161 = property on="Info" class="Str"(error in=w393, "Visible"=w383, "Text.FontBold"=w383, "Text.Text"="Populating the measurements..." ("Info")) -> (error out=w392:errorcluster)  [unwired: 1 in, 1 out]
        n162 = call "Get Measurements.vi"("Input path"=w399, "LabVIEW version"=w397, "error in (no error)"=w392) -> ("Error?"=w384:string, "VI list"=w386:T10[], "Folder list"=w385:T10[], "error out"=w398:errorcluster)  [unwired: 9 in]
        n163 = Empty String/Path?(string/path=w384) -> (empty?=w387:bool)
        n164 = case "No error occured during get measurements?" shown="True" w387 {
          tunnel: w398 -> [w400 w432]
          tunnel: w396 -> [w407 w431]
          tunnel: [w406 w430] -> w395
          tunnel: w390 -> [w405 w429]
          tunnel: [w403 w428] -> w380
          tunnel: w386 -> [_ w419]
          tunnel: w385 -> [_ w418]
          tunnel: w384 -> [w404 _]
          frame False {
            # "Update the warning"
            n165 = Bundle By Name(cluster=w407, "Tree Reference"=w405, "Measurement warning"=w404) -> (w406:T3)
            n166 = call "Queue Driver.vi"("State"="Validate inputs", "error in (no error)"=w400, "Q Operations"=Queue_Operations."Enqueue") -> ("error out"=w403:errorcluster)  [unwired: 11 in, 1 out]
          }
          frame True {
            w417 = FALSE
            # "Populate the Tree with the measurements"
            n167 = call "Populate Tree.vi"("TreeControl in"=w429, "VI list"=w419, "Folder list"=w418, "error in (no error)"=w432) -> ("TreeControl out"=w426:refnum<vi>, "error out"=w427:errorcluster)  [unwired: 10 in]
            n168 = call "Set Tree Item Icon.vi"("TreeControl in"=w426, "error in (no error)"=w427) -> ("TreeControl out"=w422:refnum<vi>, "Measurement folder Tags"=w420:string[], "Measurement file Tags"=w421:string[], "error out"=w425:errorcluster)  [unwired: 10 in]
            n169 = Empty Array?(array=w421) -> (empty?=w410:bool)
            n170 = Select(t="No Measurement found in the folder" ("Warning"), s=w410, f="Atleast one measurement should be selected" ("Text.Text")) -> (s? t:f=w411:string)
            n171 = property on="Selection warning" class="Str"(error in=w425, "Visible"=TRUE, "Text.Text"=w411) -> (error out=w416:errorcluster)  [unwired: 1 in, 1 out]
            n172 = Select(t=T4."Disabled and Grayed Out" ("Disabled"), s=w410, f=T4."Enabled") -> (s? t:f=w409:T4)
            n173 = Bundle By Name(cluster=w431, "Tree Reference"=w422, "Measurement folder Tags"=w420, "Measurement file Tags"=w421, "Select all"=w417) -> (w430:T3)
            n174 = property on="Select all" class="Bool (strict)"(error in=w416, "Value"=w417, "DisabledEnum"=w409) -> (error out=w423:errorcluster)  [unwired: 1 in, 1 out]
            n175 = property on="Tab Control" class="TabCtl (strict)"(error in=w423, "Value"=T1."Select measurements" ("Tab Control")) -> (error out=w428:errorcluster)  [unwired: 1 in, 1 out]
          }
        }
        n176 = property on="Info" class="Str"(error in=w380, "Visible"=FALSE) -> (error out=w379:errorcluster)  [unwired: 1 in, 1 out]
        n177 = call "Set Cursor Icon.vi"("Cursor icon"=u16 0, "error in (no error)"=w379) -> ("error out"=w389:errorcluster)  [unwired: 13 in]
      }
      frame "Select/Deselect all" {
        # "Update the selection of items in the Tree based on the value of Select all"
        n178 = call "Set Cursor Icon.vi"("Cursor icon"=u16 2, "error in (no error)"=w447) -> ("error out"=w436:errorcluster)  [unwired: 13 in]
        n179 = Unbundle By Name(w439) -> ("Tree Reference"=w440:refnum<vi>, "Measurement folder Tags"=w442:string[], "Measurement file Tags"=w444:string[], "Select all"=w446:bool)
        n180 = Not(x=w446) -> (.not. x?=w448:bool)
        n181 = call "Tree Icons.vi"() -> ("Not Selected"=w450:i32, "Selected"=w451:i32)  [unwired: 6 in]
        n182 = property on="Selection warning" class="Str"(error in=w436, "Text.Text"="Atleast one measurement should be selected", "Visible"=w448) -> (error out=w445:errorcluster)  [unwired: 1 in, 1 out]
        n183 = Select(t=w451, s=w446, f=w450) -> (s? t:f=w443:i32)
        n184 = call "Update Tree Item Icon.vi"("TreeControl in"=w440, "Measurement folder Tags"=w442, "Measurement file Tags"=w444, "Icon"=w443, "error in (no error)"=w445) -> ("TreeControl out"=w437:refnum<vi>, "error out"=w441:errorcluster)  [unwired: 9 in]
        n185 = Bundle By Name(cluster=w439, "Tree Reference"=w437) -> (w438:T3)
        n186 = call "Set Cursor Icon.vi"("Cursor icon"=u16 0, "error in (no error)"=w441) -> ("error out"=w435:errorcluster)  [unwired: 13 in]
      }
      frame "Measurement selection" {
        # "Update the icons of the Tree items based on the selection"
        n187 = call "Set Cursor Icon.vi"("Cursor icon"=u16 2, "error in (no error)"=w472) -> ("error out"=w457:errorcluster)  [unwired: 13 in]
        n188 = Unbundle By Name(w471) -> ("Tree Reference"=w452:refnum<vi>, "Measurement folder Tags"=w462:string[], "Measurement file Tags"=w461:string[], "Selected cell Tag"=w463:string)
        n189 = call "Update Tree Item Selection.vi"("TreeControl in"=w452, "Measurement folder Tags"=w462, "Measurement file Tags"=w461, "Selected cell Tag"=w463, "error in (no error)"=w457) -> ("TreeControl out"=w458:refnum<vi>, "error out"=w468:errorcluster)  [unwired: 9 in]
        n190 = Insert Into Array(array=w462, new element=w461) -> (w464:string[])  [unwired: 1 in]
        n191 = call "Verify Select All.vi"("TreeControl in"=w458, "Measurement Tags"=w464, "error in (no error)"=w468) -> ("TreeControl out"=w460:refnum<vi>, "Select"=w453:bool, "Deselect"=w459:bool, "error out"=w467:errorcluster)  [unwired: 9 in]
        n192 = Bundle By Name(cluster=w471, "Tree Reference"=w460, "Select all"=w453) -> (w470:T3)
        n193 = property on="Select all" class="Bool (strict)"(error in=w467, "Value"=w453) -> (error out=w466:errorcluster)  [unwired: 1 in, 1 out]
        n194 = property on="Selection warning" class="Str"(error in=w466, "Text.Text"="Atleast one measurement should be selected", "Visible"=w459) -> (error out=w469:errorcluster)  [unwired: 1 in, 1 out]
        n195 = call "Set Cursor Icon.vi"("Cursor icon"=u16 0, "error in (no error)"=w469) -> ("error out"=w455:errorcluster)  [unwired: 13 in]
      }
      frame "List plug-ins" {
        # "List the Plug-in names of the selected measurements"
        n196 = Unbundle By Name(w476) -> ("Tree Reference"=w481:refnum<vi>, "Measurement file Tags"=w487:string[], "Measurement folder selected?"=w490:bool, "Measurement file/folder path"=w489:path)
        n197 = call "Set Cursor Icon.vi"("Cursor icon"=u16 2, "error in (no error)"=w491) -> ("error out"=w480:errorcluster)  [unwired: 13 in]
        n198 = case "Measurement Folder?" shown="True" w490 {
          tunnel: w480 -> [w506 w512]
          tunnel: w489 -> [w505 _]
          tunnel: [w504 w509] -> w488
          tunnel: [w502 w508] -> w474
          tunnel: w487 -> [_ w511]
          tunnel: w481 -> [w501 w510]
          tunnel: [w501 w507] -> w473
          frame False {
            # "Get the plug-in name of the selected measurement file"
            n199 = call <vilib>:"Get File Extension.vi"("error in (no error)"=w506, "file"=w505) -> ("error out"=w504:errorcluster, "filename without extension"=w500:string)  [unwired: 5 in, 3 out]
            n200 = Build Array(w500, w500) -> (w503:string[])
            n201 = Build Array(w503) -> (w502:string[][])
          }
          frame True {
            # "Get the plug-in names of all the selected files in the measurement folder"
            n202 = call "Get Selected Measurements.vi"("Tree control in"=w510, "Measurement file Tags"=w511, "error in (no error)"=w512) -> ("Tree control out"=w507:refnum<vi>, "Measurement Plug-ins"=w508:string[][], "error out"=w509:errorcluster)  [unwired: 10 in]
          }
        }
        n203 = property on="List of Selected Measurements" class="MCListbox (strict)"(error in=w488, "ItemNames"=w474, "TopLeft"=T5 {"Row"=0, "Column"=0} ("Top Left Visible Cell")) -> (error out=w486:errorcluster)  [unwired: 1 in, 1 out]
        n204 = Bundle By Name(cluster=w476, "Tree Reference"=w473, "Measurement Plug-ins"=w474) -> (w475:T3)
        n205 = Array Size(array=w474) -> (size(s)=w484:i32[])
        n206 = Index Array(array=w484) -> (element=w483:i32)  [unwired: 1 in]
        n207 = for {
          N: w483 -> [_]
          shift-right: [w497] -> w485
          shift-left: w486 -> [w498]
          i -> [w494]
          # "Set the row size for the occupied rows"
          n208 = Bundle By Name(cluster=T6 {"Row"=0, "Column"=0} ("Active Cell:Active Cell"), "Row"=w494) -> (w496:T6)
          n209 = property on="List of Selected Measurements" class="MCListbox (strict)"(error in=w498, "ActiveCell"=w496, "Height"=u32 18 ("Active Cell:Cell Size:Height")) -> (error out=w497:errorcluster)  [unwired: 1 in, 1 out]
        }
        n210 = property on="Tab Control" class="TabCtl (strict)"(error in=w485, "Value"=T1."List Plug-ins" ("Tab Control")) -> (error out=w493:errorcluster)  [unwired: 1 in, 1 out]
        n211 = call "Set Cursor Icon.vi"("Cursor icon"=u16 0, "error in (no error)"=w493) -> ("error out"=w478:errorcluster)  [unwired: 13 in]
      }
      frame "Validate plug-in rename" {
        # "Validate the name of the Plug-in after rename"
        n212 = call "Set Cursor Icon.vi"("Cursor icon"=u16 2, "error in (no error)"=w548) -> ("error out"=w540:errorcluster)  [unwired: 13 in]
        n213 = property on="List of Selected Measurements" class="MCListbox (strict)"(error in=w540) -> (error out=w532:errorcluster, "ItemNames"=w546:string[][])  [unwired: 1 in, 1 out]
        n214 = Unbundle By Name(w544) -> ("Measurement Plug-ins"=w542:string[][], "Project path"=w530:path)
        n215 = Index Array(array=w546, index (col)=1 ("disabled index (col)")) -> (element=w515:string[])  [unwired: 1 in]
        n216 = call "Get Libraries in Project.vi"("Project path"=w530, "error in (no error)"=w532) -> ("Project exists?"=w529:bool, "Library names"=w528:string[], "error out"=w531:errorcluster)  [unwired: 11 in]
        n217 = Index Array(array=w542, index (col)=1 ("disabled index (col)")) -> (element=w514:string[])  [unwired: 1 in]
        n218 = for {
          shift-right: [w555] -> w525
          shift-left: w531 -> [w556]
          tunnel: w515 -> [w552] mode=indexing
          tunnel: w529 -> [w554]
          tunnel: w528 -> [w553]
          tunnel: [w550] -> w516 mode=indexing
          tunnel: w514 -> [w551] mode=indexing
          tunnel: [w549] -> w513 mode=indexing
          # "Validate the plug-in names"
          n219 = call "Validate Plugin Name.vi"("Project exists?"=w554, "Library names"=w553, "Plug-in name"=w552, "error in (no error)"=w556) -> ("Valid Name?"=w550:bool, "error out"=w555:errorcluster)  [unwired: 10 in]
          n220 = Swap Values(12:w551, 13:w550, 14:w552) -> (1:w549:string)  [unwired: 1 out]
        }
        n221 = call "Set Plug-in Name Warning.vi"("Valid Name?"=w516, "Validated names"=w513, "error in (no error)"=w525) -> ("Warning?"=w526:bool, "error out"=w524:errorcluster)  [unwired: 11 in]
        n222 = Replace Array Subset(array=w542, new element=w513, index (col)=1 ("disabled index (col)")) -> (w517:string[][])  [unwired: 1 in]
        n223 = property on="Plug-in warning" class="Str"(error in=w524, "Visible"=w526) -> (error out=w536:errorcluster)  [unwired: 1 in, 1 out]
        n224 = Swap Values(12:u32 250 ("Size:Height"), 13:w526, 14:210 ("x")) -> (1:w527:u32)  [unwired: 1 out]
        n225 = Bundle By Name(cluster=w544, "Measurement Plug-ins"=w517) -> (w543:T3)
        n226 = property on="List of Selected Measurements" class="MCListbox (strict)"(error in=w536, "ItemNames"=w517, "Height"=w527) -> (error out=w533:errorcluster)  [unwired: 1 in, 1 out]
        n227 = Not(x=w526) -> (.not. x?=w521:bool)
        n228 = property on="Plug-in info" class="Str"(error in=w533, "Visible"=w521) -> (error out=w523:errorcluster)  [unwired: 1 in, 1 out]
        n229 = Select(t=T4."Enabled", s=w521, f=T4."Disabled and Grayed Out" ("Disabled")) -> (s? t:f=w518:T4)
        n230 = property on="Start Migration" class="Bool"(error in=w523, "DisabledEnum"=w518) -> (error out=w522:errorcluster)  [unwired: 1 in, 1 out]
        n231 = call "Set Cursor Icon.vi"("Cursor icon"=u16 0, "error in (no error)"=w522) -> ("error out"=w538:errorcluster)  [unwired: 13 in]
      }
      frame "/**********MULTIPLE MIGRATION**********/" {
      }
      frame "Update Measurement Paths" {
        w574 = 70  # Remaining Progress
        # "Update the measurement file paths for measurement folder"
        n232 = property on="Progress" class="Slide (strict)"(error in=w564, "Value"=5 ("Progress"), "Caption.Text"="Getting paths...") -> (error out=w575:errorcluster)  [unwired: 1 in, 1 out]
        n233 = Unbundle By Name(w580) -> ("Migration Status"=w568:string[][], "Measurement Plug-ins"=w570:string[][], "Measurement file/folder path"=w583:path, "Measurement Plug-ins"=w582:string[][], "Measurement folder selected?"=w581:bool)
        n234 = property on="Measurement Count" class="Slide (strict)"(error in=w575, "Value"=0 ("Measurement Count"), "Caption.Text"="Updating Measurement Paths") -> (error out=w571:errorcluster)  [unwired: 1 in, 1 out]
        n235 = Index Array(array=w570, index (col)=1 ("disabled index (col)")) -> (element=w566:string[])  [unwired: 1 in]
        n236 = call "Get Measurement Paths.vi"("Measurement Path"=w583, "Measurement Plug-ins"=w582, "Measurement folder selected?"=w581, "error in"=w571) -> ("Measurement Path Array"=w578:path[], "error out"=w560:errorcluster)  [unwired: 10 in]
        n237 = Insert Into Array(array=w568, index (col)=0 ("disabled index (col)"), new element=w566) -> (w565:string[][])  [unwired: 1 in]
        n238 = Array Size(array=w578) -> (size(s)=w573:i32)
        n239 = Quotient & Remainder(x=w574, y=w573) -> (floor(x/y)=w572:i32)  [unwired: 1 out]
        n240 = Bundle By Name(cluster=w580, "Migration Status"=w565, "Measurement File Paths"=w578, "Plugin Migration Value"=w573, "Progress per measurement"=w572) -> (w579:T3)
        n241 = property on="Progress" class="Slide (strict)"(error in=w560, "Value"=15 ("Progress")) -> (error out=w559:errorcluster)  [unwired: 1 in, 1 out]
      }
      frame "Create Project" {
        # "Check if project exists and creates a new project if not present."
        n242 = property on="Progress" class="Slide (strict)"(error in=w587, "Value"=10 ("Progress"), "Caption.Text"="Checking for project...") -> (error out=w588:errorcluster)  [unwired: 1 in, 1 out]
        n243 = property on="Measurement Count" class="Slide (strict)"(error in=w588, "Value"=10 ("Measurement Count"), "Caption.Text"="Creating project if not exist") -> (error out=w591:errorcluster)  [unwired: 1 in, 1 out]
        n244 = Unbundle By Name(w595) -> ("Project path"=w594:path)
        n245 = call "Create and Save Project.vi"("Project Path"=w594, "error in (no error)"=w591) -> ("error out"=w585:errorcluster)  [unwired: 13 in]
        n246 = property on="Progress" class="Slide (strict)"(error in=w585, "Value"=15 ("Progress")) -> (error out=w584:errorcluster)  [unwired: 1 in, 1 out]
      }
      frame "Migrate measurements" {
        # "Migrate multiple measurements along with their shared dependencies"
        n247 = property on="Progress" class="Slide (strict)"(error in=w597, "Value"=0 ("Progress")) -> (error out=w598:errorcluster)  [unwired: 1 in, 1 out]
        n248 = Unbundle By Name(w608) -> ("Project path"=w612:path, "Measurement File Paths"=w610:path[], "Measurement Plug-ins"=w613:string[][])
        n249 = property on="Measurement Count" class="Slide (strict)"(error in=w598, "Value"=20 ("Measurement Count"), "Caption.Text"="Migrating measurement(s)") -> (error out=w603:errorcluster)  [unwired: 1 in, 1 out]
        n250 = Index Array(array=w613, index (col)=1 ("disabled index (col)")) -> (element=w611:string[])  [unwired: 1 in]
        n251 = control-ref of="Progress"() -> (w596:refnum<vi>)
        n252 = call "Migrate Dependencies.vi"("Project path"=w612, "Measurement paths"=w610, "Plug-in names"=w611, "Progress"=w596, "error in"=w603) -> ("Instrument containing subVIs"=w607:path[][], "error out"=w601:errorcluster)  [unwired: 9 in]
        n253 = Bundle By Name(cluster=w608, "Instrument containing subVIs"=w607, "Measurement Progress"=30) -> (w609:T3)
        n254 = property on="Measurement Count" class="Slide (strict)"(error in=w601, "Value"=30 ("Measurement Count")) -> (error out=w600:errorcluster)  [unwired: 1 in, 1 out]
      }
      frame "Enqueue Migration Steps" {
        # "Enqueue the set of states for measurement migration"
        n255 = Unbundle By Name(w619) -> ("Plugin Migration Value"=w618:i32)
        n256 = Greater Than 0?(x=w618) -> (x > 0?=w617:bool)
        n257 = case shown="True" w617 {
          tunnel: w616 -> [w622 w629]
          tunnel: [w624 w628] -> w615
          frame False {
            # "Enqueue next step if all measurements are migrated"
            n258 = property on="Measurement Count" class="Slide (strict)"(error in=w622, "Value"=100 ("Progress")) -> (error out=w623:errorcluster)  [unwired: 1 in, 1 out]
            n259 = call "Queue Driver.vi"("States[]"=string[] ["Save Project", "Show Next Steps"], "error in (no error)"=w623, "Q Operations"=Queue_Operations."Enqueue N") -> ("error out"=w624:errorcluster)  [unwired: 11 in, 1 out]
          }
          frame True {
            # "Enqueue, if there are measurements yet to migrate"
            n260 = call "Queue Driver.vi"("States[]"=string[] ["Set Values in Dict", "Create Plugin Template", "Get Driver List", "Edit Measurement Configuration", "Edit Measurement Results", "Edit Measurement Connector Pane", "Create Wrapper", "Deserialize Cluster Data", "Add Measurement Plugin APIs", "Disable Initialize APIs", "Edit Type Specialization", "Add UI Elements", "Flatten the Clusters", "Handling Default Value", "Update Migration Count"], "error in (no error)"=w629, "Q Operations"=Queue_Operations."Enqueue N") -> ("error out"=w628:errorcluster)  [unwired: 11 in, 1 out]
          }
        }
      }
      frame "Set Values in Dict" {
        # "Measurement Status Message: Migrating 1 of N measurement(s)"
        # "Set values to the Dictionary APIs"
        n261 = Unbundle By Name(w652) -> ("Project path"=w646:path, "Instrument containing subVIs"=w642:path[][], "Measurement Plug-ins"=w651:string[][], "Migration Count"=w630:i32, "Measurement File Paths"=w639:path[])
        n262 = property on="Progress" class="Slide (strict)"(error in=w633, "Value"=0 ("Progress")) -> (error out=w638:errorcluster)  [unwired: 1 in, 1 out]
        n263 = Array Size(array=w639) -> (size(s)=w631:i32)
        n264 = Increment(x=w630) -> (x+1=w635:i32)
        n265 = Format Into String(format string="Migrating %d of %d measurement(s)", error in=w638, w635, w631) -> (resulting string=w636:string, error out=w637:errorcluster)  [unwired: 1 in]
        n266 = property on="Measurement Count" class="Slide (strict)"(error in=w637, "Caption.Text"=w636) -> (error out=w640:errorcluster)  [unwired: 1 in, 1 out]
        n267 = Index Array(array=w639, index=w630) -> (element=w649:path)
        n268 = call "Set Code Module Path.vi"("CodeModule Path"=w649, "error in (no error)"=w640) -> ("error out"=w648:errorcluster)  [unwired: 13 in]
        n269 = Index Array(array=w651, index (row)=w630, index (col)=1 ("disabled index (col)")) -> (element=w647:string)
        n270 = Index Array(array=w642, index (row)=w630) -> (element=w645:path[])  [unwired: 1 in]
        n271 = call "Set Measurement Name.vi"("Name"=w647, "error in (no error)"=w648) -> ("error out"=w644:errorcluster)  [unwired: 13 in]
        n272 = call "Set Instrument VI Paths.vi"("error in (no error)"=w644, "VI Paths[]"=w645) -> ("error out"=w643:errorcluster)  [unwired: 9 in]
        n273 = call "Set Project Path.vi"("Project Path"=w646, "error in (no error)"=w643) -> ("error out"=w632:errorcluster)  [unwired: 13 in]
      }
      frame "Create Plugin Template" {
        # "Create Measurement Plugin Template"
        n274 = property on="Progress" class="Slide (strict)"(error in=w655, "Value"=1 ("Progress"), "Caption.Text"="Creating Measurement Plugin...") -> (error out=w656:errorcluster)  [unwired: 1 in, 1 out]
        n275 = Unbundle By Name(w660) -> ("Project path"=w659:path)
        n276 = call "Create Plugin Template.vi"("Project Path"=w659, "error in (no error)"=w656) -> ("error out"=w658:errorcluster)  [unwired: 13 in]
        n277 = call "Copy Set Default Value Multiple.vi"("error in (no error)"=w658) -> ("error out"=w654:errorcluster)  [unwired: 14 in]
      }
      frame "Get Driver List" {
        # "Get the list of instrument drivers used in the measurement"
        n278 = property on="Progress" class="Slide (strict)"(error in=w662, "Value"=3 ("Progress"), "Caption.Text"="Fetching the list of instrument drivers used...") -> (error out=w663:errorcluster)  [unwired: 1 in, 1 out]
        n279 = call "List Drivers.vi"("error in (no error)"=w663) -> ("error out"=w664:errorcluster)  [unwired: 14 in]
      }
      frame "Edit Measurement Configuration" {
        # "Add elements to the measurement configuration control file"
        n280 = property on="Progress" class="Slide (strict)"(error in=w668, "Value"=4 ("Progress"), "Caption.Text"="Editing measurement configuration...") -> (error out=w669:errorcluster)  [unwired: 1 in, 1 out]
        n281 = call "Add Measurement Plugin Controls.vi"("error in (no error)"=w669) -> ("error out"=w670:errorcluster)  [unwired: 14 in]
      }
      frame "Edit Measurement Results" {
        # "Add elements to the measurement results control file"
        n282 = property on="Progress" class="Slide (strict)"(error in=w674, "Value"=5 ("Progress"), "Caption.Text"="Editing measurement results...") -> (error out=w675:errorcluster)  [unwired: 1 in, 1 out]
        n283 = call "Add Meas Plugin Indicators.vi"("error in (no error)"=w675) -> ("error out"=w676:errorcluster)  [unwired: 14 in]
      }
      frame "Edit Measurement Connector Pane" {
        # "Edit the connector pane of the duplicated measurement"
        n284 = property on="Progress" class="Slide (strict)"(error in=w680, "Value"=6 ("Progress"), "Caption.Text"="Editing the connector pane of the measurement...") -> (error out=w681:errorcluster)  [unwired: 1 in, 1 out]
        n285 = call "Edit Connector Pane Multiple.vi"("error in (no error)"=w681) -> ("error out"=w682:errorcluster)  [unwired: 14 in]
      }
      frame "Create Wrapper" {
        # "Create a wrapper for the measurement"
        n286 = property on="Progress" class="Slide (strict)"(error in=w686, "Value"=7 ("Progress"), "Caption.Text"="Creating wrapper for the measurement...") -> (error out=w687:errorcluster)  [unwired: 1 in, 1 out]
        n287 = call "Create Wrapper for Measurement Plugin.vi"("error in (no error)"=w687) -> ("error out"=w688:errorcluster)  [unwired: 14 in]
      }
      frame "Deserialize Cluster Data" {
        # "Deserialize the connection in the wrapper vi"
        n288 = property on="Progress" class="Slide (strict)"(error in=w692, "Value"=8 ("Progress"), "Caption.Text"="Flattening and unflattening the cluster data in Wrapper...") -> (error out=w693:errorcluster)  [unwired: 1 in, 1 out]
        n289 = call "Deserialize Connections in Wrapper Plugin.vi"("error in (no error)"=w693) -> ("error out"=w694:errorcluster)  [unwired: 14 in]
      }
      frame "Add Measurement Plugin APIs" {
        # "Add all the rquired Measurement Plugin APIs in measurement logic and wire them appropriately"
        n290 = property on="Progress" class="Slide (strict)"(error in=w698, "Value"=9 ("Progress"), "Caption.Text"="Editing measurement logic...") -> (error out=w699:errorcluster)  [unwired: 1 in, 1 out]
        n291 = call "Create Measurement Plugin subVIs.vi"("error in (no error)"=w699) -> ("error out"=w700:errorcluster)  [unwired: 14 in]
      }
      frame "Disable Initialize APIs" {
        # "Disable the initialize and close in the measurement"
        n292 = property on="Progress" class="Slide (strict)"(error in=w704, "Value"=10 ("Progress"), "Caption.Text"="Disabling and removing the Initalize and Close APIs...") -> (error out=w705:errorcluster)  [unwired: 1 in, 1 out]
        n293 = call "Add Diagram disable structure.vi"("error in (no error)"=w705) -> ("error out"=w706:errorcluster)  [unwired: 14 in]
      }
      frame "Edit Type Specialization" {
        # "Edit the Type Specializations.vi"
        n294 = property on="Progress" class="Slide (strict)"(error in=w710, "Value"=11 ("Progress"), "Caption.Text"="Editing the Type Specialization VI...") -> (error out=w711:errorcluster)  [unwired: 1 in, 1 out]
        n295 = call "Edit Plugin Type Specialization.vi"("error in (no error)"=w711) -> ("error out"=w712:errorcluster)  [unwired: 14 in]
      }
      frame "Add UI Elements" {
        # "Edit the Measurement UI.vi"
        n296 = property on="Progress" class="Slide (strict)"(error in=w716, "Value"=12 ("Progress"), "Caption.Text"="Editing Measurement UI...") -> (error out=w717:errorcluster)  [unwired: 1 in, 1 out]
        n297 = call "Add Elements to Meas Plugin UI.vi"("error in (no error)"=w717) -> ("error out"=w718:errorcluster)  [unwired: 14 in]
      }
      frame "Flatten the Clusters" {
        # "Creating string ande serialize data for the wrapper connections"
        n298 = property on="Progress" class="Slide (strict)"(error in=w722, "Value"=13 ("Progress"), "Caption.Text"="Creating events and flatten the data...") -> (error out=w723:errorcluster)  [unwired: 1 in, 1 out]
        n299 = call "Create String and Serialize Cluster Data in UI.vi"("error in (no error)"=w723) -> ("error out"=w724:errorcluster)  [unwired: 14 in]
      }
      frame "Handling Default Value" {
        # "Setting default value for cluster based on string controls"
        n300 = property on="Progress" class="Slide (strict)"(error in=w728, "Value"=14 ("Progress"), "Caption.Text"="Loading values for string controls in UI...") -> (error out=w729:errorcluster)  [unwired: 1 in, 1 out]
        n301 = call "Logic for Default Case Multiple.vi"("error in (no error)"=w729) -> ("error out"=w730:errorcluster)  [unwired: 14 in]
      }
      frame "Save Project" {
        # "Saving the project and libraries"
        n302 = property on="Progress" class="Slide (strict)"(error in=w734, "Value"=15 ("Progress"), "Caption.Text"="Saving the project files...") -> (error out=w736:errorcluster)  [unwired: 1 in, 1 out]
        n303 = call "Save Projects and Libraries.vi"("error in (no error)"=w736) -> ("error out"=w735:errorcluster)  [unwired: 10 in]
      }
      frame "Update Migration Count" {
        # "Updating the migration count and migration status"
        n304 = in-place {
          in-place-border: [w747] -> w741
          n305 = in-place-cluster #2(w746) -> ("Plugin Migration Value"=w759:i32, "Migration Count"=w750:i32, "Measurement Progress"=w757:i32, "Progress per measurement"=w756:i32, "Migration Status"=w753:string[][])
          n306 = Index Array(array=w753, index (col)=1 ("disabled index (col)")) -> (element=w751:string[])  [unwired: 1 in]
          n307 = Insert Into Array(array=w751, index=w750, new element="Success") -> (w748:string[])
          n308 = Insert Into Array(array=w753, index (col)=1 ("disabled index (col)"), new element=w748) -> (w755:string[][])  [unwired: 1 in]
          n309 = Increment(x=w750) -> (x+1=w760:i32)
          n310 = Add(x=w757, y=w756) -> (x+y=w747:i32)
          n311 = Decrement(x=w759) -> (x-1=w758:i32)
          n312 = in-place-cluster #2("Plugin Migration Value"=w758, "Migration Count"=w760, "Measurement Progress"=w747, "Progress per measurement"=w756, "Migration Status"=w755) -> (w745:T3)
        }
        n313 = property on="Measurement Count" class="Slide (strict)"(error in=w740, "Value"=w741) -> (error out=w739:errorcluster)  [unwired: 1 in, 1 out]
        n314 = call "Queue Driver.vi"("State"="Enqueue Migration Steps", "error in (no error)"=w739, "Q Operations"=Queue_Operations."Enqueue") -> ("error out"=w744:errorcluster)  [unwired: 11 in, 1 out]
      }
      frame "Update count on Fail" {
        # "Updating the migration count and migration status"
        n315 = in-place {
          in-place-border: [w769] -> w763
          n316 = in-place-cluster #3(w768) -> ("Plugin Migration Value"=w781:i32, "Migration Count"=w772:i32, "Measurement Progress"=w779:i32, "Progress per measurement"=w778:i32, "Migration Status"=w775:string[][])
          n317 = Index Array(array=w775, index (col)=1 ("disabled index (col)")) -> (element=w773:string[])  [unwired: 1 in]
          n318 = Insert Into Array(array=w773, index=w772, new element="Fail") -> (w770:string[])
          n319 = Insert Into Array(array=w775, index (col)=1 ("disabled index (col)"), new element=w770) -> (w777:string[][])  [unwired: 1 in]
          n320 = Increment(x=w772) -> (x+1=w782:i32)
          n321 = Add(x=w779, y=w778) -> (x+y=w769:i32)
          n322 = Decrement(x=w781) -> (x-1=w780:i32)
          n323 = in-place-cluster #3("Plugin Migration Value"=w780, "Migration Count"=w782, "Measurement Progress"=w769, "Progress per measurement"=w778, "Migration Status"=w777) -> (w767:T3)
        }
        n324 = property on="Measurement Count" class="Slide (strict)"(error in=w762, "Value"=w763) -> (error out=w761:errorcluster)  [unwired: 1 in, 1 out]
        n325 = call "Queue Driver.vi"("State"="Enqueue Migration Steps", "error in (no error)"=w761, "Q Operations"=Queue_Operations."Enqueue") -> ("error out"=w766:errorcluster)  [unwired: 11 in, 1 out]
      }
      frame "/**********NEXT STEPS POST MIGRATION**********/" {
      }
      frame "Show Next Steps" {
        # "To change unwanted loading symbol"
        # "Showing the migration status"
        n326 = in-place {
          in-place-border: [w808] -> w792
          n327 = in-place-cluster #4(w800) -> ("Migration Status"=w809:string[][])
          n328 = Index Array(array=w809, index (col) #1=0 ("disabled index (col)"), index (col) #2=1 ("index (col)")) -> (element #1=w812:string[], element #2=w810:string[])  [unwired: 2 in]
          n329 = for {
            tunnel: w812 -> [_] mode=indexing
            tunnel: w810 -> [w819]
            shift-right: [w814] -> w808
            shift-left: w809 -> [w817]
            i -> [w816]
            n330 = Index Array(array=w819, index=w816) -> (element=w818:string)
            n331 = Empty String/Path?(string/path=w818) -> (empty?=w815:bool)
            n332 = case shown="True" w815 {
              tunnel: w817 -> [w820 w827]
              tunnel: w816 -> [_ w824]
              tunnel: [w820 w828] -> w814
              frame False {
              }
              frame True {
                # "Insert 'Fail' for empty status"
                n333 = Index Array(array=w827, index (col)=1 ("disabled index (col)")) -> (element=w825:string[])  [unwired: 1 in]
                n334 = Insert Into Array(array=w825, index=w824, new element="Fail" ("new element/subarray")) -> (w822:string[])
                n335 = Insert Into Array(array=w827, index (col)=1 ("disabled index (col)"), new element=w822) -> (w828:string[][])  [unwired: 1 in]
              }
            }
          }
          n336 = in-place-cluster #4("Migration Status"=w808) -> (w799:T3)
        }
        n337 = property on="Tab Control" class="TabCtl (strict)"(error in=w795, "Value"=T1."Status" ("Tab Control")) -> (error out=w797:errorcluster)  [unwired: 1 in, 1 out]
        n338 = property on="Migration Status" class="MCListbox (strict)"(error in=w797, "Allow Editing Cells"=FALSE) -> (error out=w796:errorcluster)  [unwired: 1 in, 1 out]
        n339 = property on="Migration Status" class="MCListbox (strict)"(error in=w796, "ItemNames"=w792) -> (error out=w787:errorcluster)  [unwired: 1 in, 1 out]
        n340 = Index Array(array=w792, index (col)=1 ("disabled index (col)")) -> (element=w790:string[])  [unwired: 1 in]
        n341 = Equal?(x=w790, y="Fail" ("new element/subarray")) -> (x = y?=w788:bool[])
        n342 = And Array Elements(Boolean array=w788) -> (logical AND=w785:bool)
        n343 = case "All the measurements failed?" shown="True" w785 {
          tunnel: w787 -> [w803 w807]
          tunnel: [w804 w806] -> w786
          frame False {
            n344 = property on="Review" class="Bool"(error in=w803, "BoolText.Text"="Review Plug-ins" ("Boolean Text.Text")) -> (error out=w804:errorcluster)  [unwired: 1 in, 1 out]
          }
          frame True {
            # "Change Bool Text to Start next migration"
            n345 = property on="Review" class="Bool"(error in=w807, "BoolText.Text"="Start Next Migration" ("Boolean Text.Text")) -> (error out=w806:errorcluster)  [unwired: 1 in, 1 out]
          }
        }
        n346 = call "Set Cursor Icon.vi"("Cursor icon"=u16 0, "error in (no error)"=w786) -> ("error out"=w794:errorcluster)  [unwired: 13 in]
      }
      frame "Show Links" {
        # "Showing links for the migrated measurements"
        n347 = Unbundle By Name(w836) -> ("Migration Status"=w838:string[][])
        n348 = for {
          tunnel: w838 -> [w845] mode=indexing
          tunnel: [w839] -> w833 mode=indexing if=w842
          # "Populating combo box with successfully migrated plugin names"
          n349 = Index Array(array=w845, index #1=0 ("index"), index #2=1 ("index")) -> (element #1=w839:string, element #2=w840:string)
          n350 = Equal?(x=w840, y="Success") -> (x = y?=w842:bool)
        }
        n351 = Index Array(array=w833, index=0) -> (element=w829:string)
        n352 = property on="Select Plug-in" class="CmbBox"(error in=w837, "Strings[]"=w833, "Value"=w829) -> (error out=w831:errorcluster)  [unwired: 1 in, 1 out]
        n353 = call "Set Measurement Name.vi"("Name"=w829, "error in (no error)"=w831) -> ("error out"=w830:errorcluster)  [unwired: 13 in]
        n354 = property on="Tab Control" class="TabCtl (strict)"(error in=w830, "Value"=T1."Links" ("Tab Control")) -> (error out=w834:errorcluster)  [unwired: 1 in, 1 out]
      }
      frame "/**********ERROR**********/" {
      }
      frame "Error" {
        # "Handle the error and alert user"
        n355 = call <vilib>:"Clear Errors.vi"("error in (no error)"=w855) -> ("error out"=w856:errorcluster)  [unwired: 5 in, 1 out]
        n356 = Equal?(x=string[] ["Set Values in Dict", "Create Plugin Template", "Get Driver List", "Edit Measurement Configuration", "Edit Measurement Results", "Edit Measurement Connector Pane", "Create Wrapper", "Deserialize Cluster Data", "Add Measurement Plugin APIs", "Disable Initialize APIs", "Edit Type Specialization", "Add UI Elements", "Flatten the Clusters", "Handling Default Value", "Update Migration Count"] ("States[]"), y=w848) -> (x = y?=w850:bool[])
        n357 = call "Queue Driver.vi"("error in (no error)"=w856, "Q Operations"=Queue_Operations."Flush") -> ("error out"=w853:errorcluster)  [unwired: 12 in, 1 out]
        n358 = Or Array Elements(Boolean array=w850) -> (logical OR=w849:bool)
        n359 = case shown="True" w849 {
          tunnel: w853 -> [w863 w875]
          tunnel: [w862 w873] -> w852
          tunnel: w848 -> [w861 _]
          frame False {
            # "If error occurs in other steps"
            n360 = Equal?(x=string[] ["Update Measurement Paths", "Create Project", "Migrate measurements"] ("States[]"), y=w861) -> (x = y?=w859:bool[])
            n361 = Or Array Elements(Boolean array=w859) -> (logical OR=w858:bool)
            n362 = case "Error in Migration?" shown="False" w858 {
              tunnel: w863 -> [w867 w870]
              tunnel: [w866 w869] -> w862
              frame False {
                # "Restart Migration tool"
                n363 = call "Queue Driver.vi"("States[]"=string[] ["Reinitialize", "Initialize UI", "Populate project path"], "error in (no error)"=w867, "Q Operations"=Queue_Operations."Enqueue N") -> ("error out"=w866:errorcluster)  [unwired: 11 in, 1 out]
              }
              frame True {
                # "Show Next steps"
                n364 = call "Queue Driver.vi"("State"="Show Next Steps", "error in (no error)"=w870, "Q Operations"=Queue_Operations."Enqueue") -> ("error out"=w869:errorcluster)  [unwired: 11 in, 1 out]
              }
            }
          }
          frame True {
            # "If error occurs during measurement migration"
            n365 = call "Queue Driver.vi"("State"="Update count on Fail", "error in (no error)"=w875, "Q Operations"=Queue_Operations."Enqueue") -> ("error out"=w873:errorcluster)  [unwired: 11 in, 1 out]
          }
        }
      }
      frame "/**********EXIT**********/" {
      }
      frame "Exit" {
        # "Flush the queue elements and stop execution"
        n366 = call "Queue Driver.vi"("error in (no error)"=w888, "Q Operations"=Queue_Operations."Flush") -> ("error out"=w882:errorcluster)  [unwired: 12 in, 1 out]
        n367 = call "Queue Driver.vi"("error in (no error)"=w882, "Q Operations"=Queue_Operations."Release") -> ("error out"=w881:errorcluster)  [unwired: 12 in, 1 out]
        n368 = Unbundle By Name(w886) -> ("Tree Reference"=w885:refnum<vi>)
        n369 = Close Reference(reference=w885, error in (no error)=w881) -> (error out=w879:errorcluster)
        n370 = call "Dictionary.vi"("error in (no error)"=w879, "Dict States"=Dictionary_States."Delete All") -> ("error out"=w878:errorcluster)  [unwired: 12 in, 1 out]
      }
    }
  }
  n371 = invoke class="VI" method="FP.Close"(error in=w6) -> (error out=→"error out":errorcluster)  [unwired: 2 in, 2 out]
